vi "Event Handler.vi"(0 "uService Template in":refnum<class "New uService Template.lvclass">, 5 "Event type":T1=enum."Message", 7 "Item Name":string, 9 "Data":variant, 11 "error in (no error)":errorcluster) -> (4 "uService Template out":refnum<class "New uService Template.lvclass">, 15 "error out":errorcluster)   [LabVIEW 2021, in "New uService Template.lvlib" / "New uService Template.lvclass"]
doc: "This VI is the event handler of the uService: every time an event is triggered to the uService, this VI is called.\nNote: here you can access the Actor/Class data, but it will be the one coming out from Init. You cannot modify the values.\nThree different events are supported:\nI) Button Pressed: get called on a GUI button pressed. Item Name is the name (label) of the button, Data is empty.\nII) Shared Variable Updated: get called when a SV you subscribed to is updated. Item Name is the name of the SV, and Data is the value (note: you need to convert it to the proper type).\nIII) Message: get called every time a user event is generated using Send Message to Event Handler. The values of Item Name and Data are the one given to the Send Message to Event Handler.\nIV) Ready to launch?: this frame get called every time a new Run is initiated. Each uService is responsible of performing a self check before giving back the green light for the Run to start."
uses:
  New uService Template.lvclass
  TALOS/TALOS_PPL.lvlibp
  C:/LabVIEW Code/aegis-labview-code/TALOS/TALOS_PPL.lvlibp/Father of all uServices/Father of all uServices/Father of all uServices.lvclass
  C:/LabVIEW Code/aegis-labview-code/TALOS/TALOS_PPL.lvlibp/Ancestor/Ancestor/Ancestor.lvclass
  C:/LabVIEW Code/aegis-labview-code/TALOS/Actor Framework.lvlibp/1abvi3w/vi.lib/ActorFramework/Actor/Actor.lvclass
  C:/LabVIEW Code/aegis-labview-code/Other uServices/New uService Template/New uService Template.lvclass
  TALOS/TALOS_PPL.lvlibp/Father of all uServices/Father of all uServices/Father of all uServices.lvclass
  Consumer Case Selector.ctl
  TALOS/TALOS_PPL.lvlibp/Father of all uServices/Father of all uServices/Event Handler Items.ctl
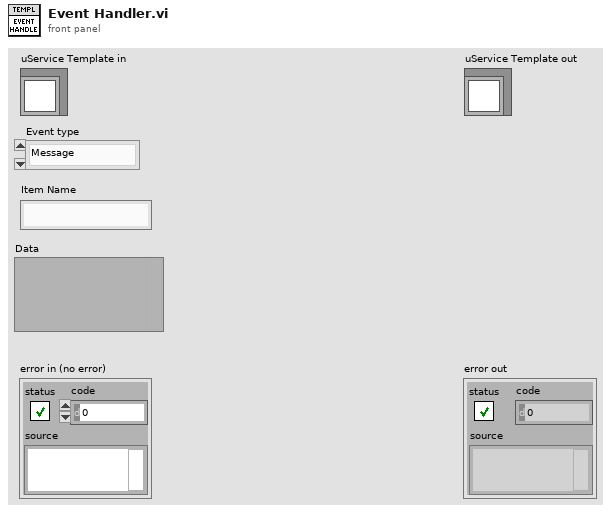
[diagram p1: front panel]
types:
  T1 = typedef "TALOS_PPL.lvlibp/Father of all uServices.lvlib/Father of all uServices.lvclass/Event Handler Items.ctl" = enum16{"Button Pressed", "Message", "Ready to launch?", "Safe Mode", "Start RUN", "Stop RUN"}
  T2 = typedef "New uService Template.lvlib/New uService Template.lvclass/Consumer Case Selector.ctl" = enum16{"Example"}
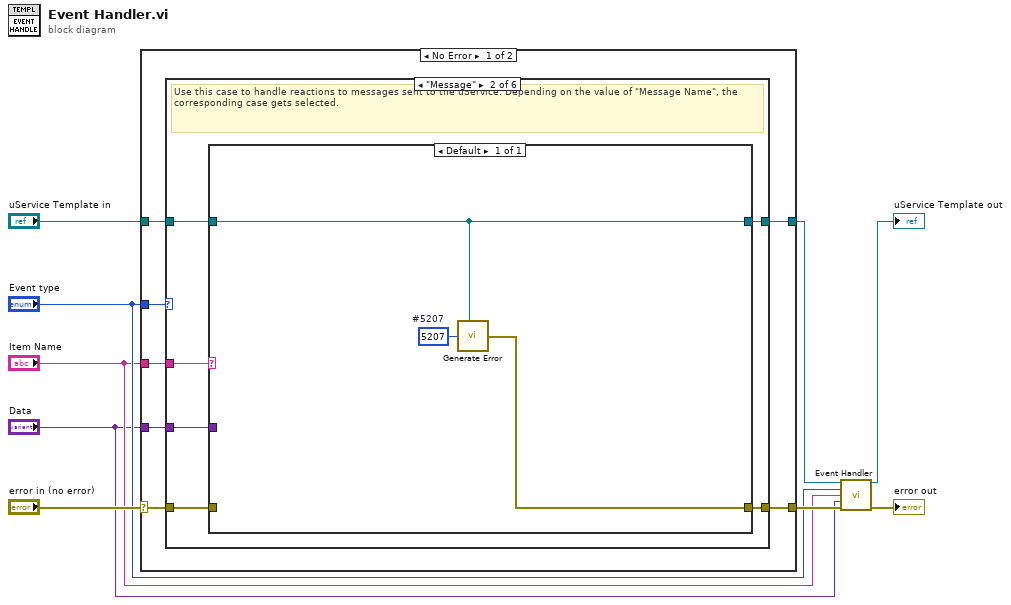
[diagram p0: block diagram]
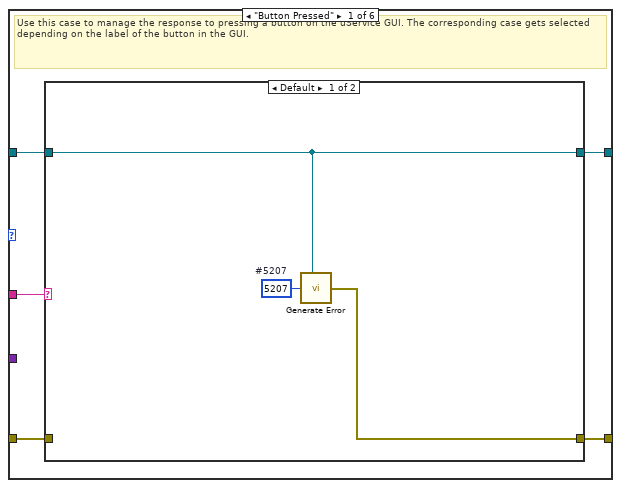
[diagram p2: hidden frame]
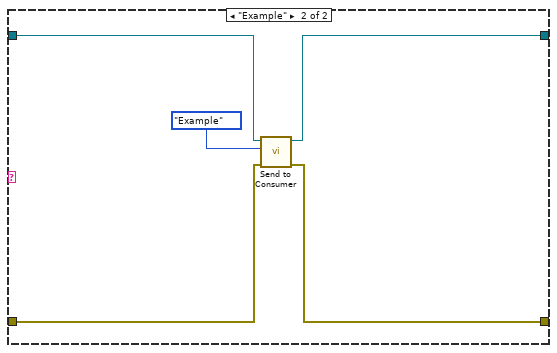
[diagram p3: hidden frame]
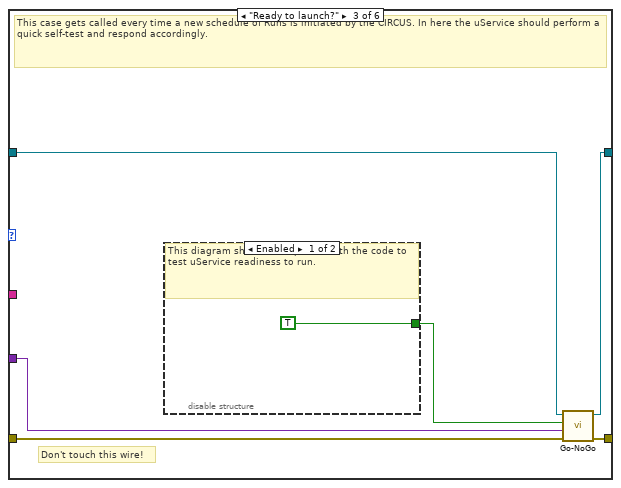
[diagram p4: hidden frame]
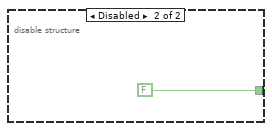
[diagram p5: hidden frame]
diagram:
  n1 = case shown="No Error" "error in (no error)" {
    selector: "error in (no error)" -> [w14 w54]
    tunnel: [w15 w54] -> w7
    tunnel: [w10 w53] -> w4
    tunnel: "uService Template in" -> [w13 w53]
    tunnel: "Event type" -> [w16 _]
    tunnel: "Item Name" -> [w12 _]
    tunnel: "Data" -> [w11 _]
    frame No Error {
      n2 = case shown="\"Message\"" w16 {
        tunnel: [w21 w31 w43 w48 w50 w52] -> w15
        tunnel: w14 -> [w18 w35 w44 w48 w50 w52]
        tunnel: w12 -> [w19 w34 _ _ _ _]
        tunnel: w13 -> [w20 w32 w42 w47 w49 w51]
        tunnel: w11 -> [_ w33 w40 _ _ _]
        tunnel: [w17 w30 w39 w47 w49 w51] -> w10
        frame "Button Pressed" {
          # "Use this case to manage the response to pressing a button on the uService GUI. The corresponding case gets selected depending on the label of the button in the GUI."
          n3 = case shown="Default" w19 {
            tunnel: w18 -> [_ w28]
            tunnel: [w23 w29] -> w21
            tunnel: w20 -> [w22 w26]
            tunnel: [w22 w25] -> w17
            frame Default {
              w24 = 5207  # #5207
              n4 = call "Generate Error.vi"("Class"=w22, "Error Code"=w24) -> ("error out"=w23:errorcluster)  [unwired: 5 in]
            }
            frame "Example" {
              n5 = call "Send to Consumer.vi"("error in (no error)"=w28, "Case ID"=Consumer_Case_Selector."Example" ("Consumer Case Selector"), "uService Template in"=w26) -> ("error out"=w29:errorcluster, "uService Template out"=w25:refnum<class "New uService Template.lvclass">)  [unwired: 7 in]
            }
          }
        }
        frame "Message" {
          # "Use this case to handle reactions to messages sent to the uService. Depending on the value of \"Message Name\", the corresponding case gets selected."
          n6 = case shown="Default" w34 {
            tunnel: w35 -> [_]
            tunnel: w33 -> [_]
            tunnel: w32 -> [w36]
            tunnel: [w37] -> w31
            tunnel: [w36] -> w30
            frame Default {
              w38 = 5207  # #5207
              n7 = call "Generate Error.vi"("Class"=w36, "Error Code"=w38) -> ("error out"=w37:errorcluster)  [unwired: 5 in]
            }
          }
        }
        frame "Ready to launch?" {
          # "Don't touch this wire!"
          # "This case gets called every time a new schedule of Runs is initiated by the CIRCUS. In here the uService should perform a quick self-test and respond accordingly."
          n8 = disable-structure shown="Enabled" {
            disable-tunnel: [TRUE ("Go?") FALSE ("Go?")] -> w41
            frame Enabled {
              # "This diagram should be replaced with the code to test uService readiness to run."
            }
            frame Disabled {
            }
          }
          n9 = call-dynamic "Go-NoGo.vi"("error in (no error)"=w44, "Go-NoGo Data"=w40, "Go?"=w41, "Father of all uServices in"=w42) -> ("error out"=w43:errorcluster, "Father of all uServices out"=w39:refnum<class "New uService Template.lvclass">)  [unwired: 6 in]
        }
        frame "Safe Mode" {
          # "This case gets triggered when Safe Mode is raised. The uService should be safely put in an idle state here."
        }
        frame "Start RUN" {
          # "This case gets triggered when a new script is launcher."
        }
        frame "Stop RUN" {
          # "This case is called whenever a script has finished execution."
        }
      }
    }
    frame Error {
    }
  }
  n10 = call-parent "Event Handler.vi"("uService Template in"=w4, "Event type"="Event type", "Item Name"="Item Name", "Data"="Data", "error in (no error)"=w7) -> ("uService Template out"=→"uService Template out":refnum<class "New uService Template.lvclass">, "error out"=→"error out":errorcluster)  [unwired: 9 in]
